vi "frequency to gpib command.vi"(1 "Input Frequency":dbl=45000000.0 min=0.5960000157356262 max=320000000.0 step=1000.0 format="%.4e") -> (0 "Final GPIB Command":string)   [LabVIEW 2022 SP3]
panel:
  out "Output string":string[](array[string])
  in  "?":i32[](array[numeric])=[8, 4, 2, 1] min=0
  out "?":i32[](array[numeric]) min=0 max=1
  out "Output String":i32[](array[numeric]) min=0 max=1
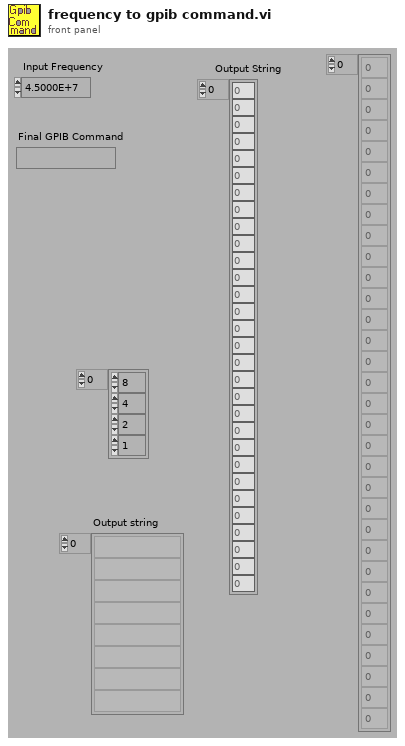
[diagram p1: front panel]
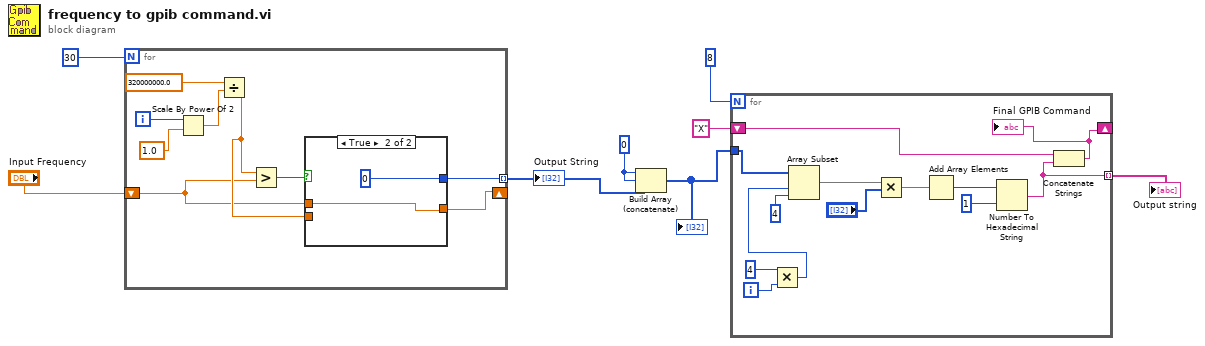
[diagram p0: block diagram]
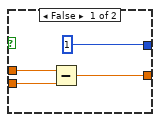
[diagram p2: hidden frame]
diagram:
  w4 = 0
  n1 = for {
    N: i8 30 -> [_]
    tunnel: [w11] -> w5 mode=indexing
    shift-right: [w9] -> _
    shift-left: "Input Frequency" -> [w10]
    i -> [w17]
    n2 = Scale By Power Of 2(n=w17, x=sgl[unit] 1.0 ("?")) -> (x*2^n=w15:sgl[unit])
    n3 = Divide(x=dbl[unit] 320000000.0 ("?"), y=w15) -> (x/y=w12:dbl)
    n4 = Greater?(x=w12, y=w10) -> (0:w13:bool)
    n5 = case shown="True" w13 {
      tunnel: w12 -> [w21 _]
      tunnel: [1 0] -> w11
      tunnel: w10 -> [w19 w22]
      tunnel: [w18 w22] -> w9
      frame False {
        n6 = Subtract(x=w19, y=w21) -> (x-y=w18:dbl)
      }
      frame True {
      }
    }
  }
  "Output String" <- w5
  n7 = Build Array (concatenate)(w4, w4, w5) -> (w3:i32[])
  "?" <- w3
  n8 = for {
    N: 8 -> [_]
    tunnel: w3 -> [w35]
    tunnel: [w25] -> w2 mode=indexing
    shift-right: [w24] -> _
    shift-left: "X" -> [w26]
    i -> [w31]
    n9 = Multiply(x=4, y=w31) -> (x*y=w30:i32)
    n10 = Array Subset(array=w35, index=w30, length=4) -> (w34:i32[])
    n11 = Multiply(x=w34, y="?") -> (x*y=w29:i32[])
    n12 = Add Array Elements(numeric array=w29) -> (sum=w28:i32)
    n13 = Number To Hexadecimal String(1:1, 2:w28) -> (0:w25:string)
    n14 = Concatenate Strings(w26, w25) -> (w24:string)
    "Final GPIB Command" <- w24
  }
  "Output string" <- w2
